vi "Write Sample Time.vi"(8 "error in (no error)":errorcluster, 10 "Sample Time":i32=1000, 11 "SensorInfo in":refnum<class "SensorInfo.lvclass">) -> (0 "error out":errorcluster, 3 "SensorInfo out":refnum<class "SensorInfo.lvclass">)   [LabVIEW 2012, in "Sensor Definition.lvlib" / "SensorInfo.lvclass"]
uses:
  SensorInfo.lvclass
  SensorInfo.lvclass/SensorInfo.ctl
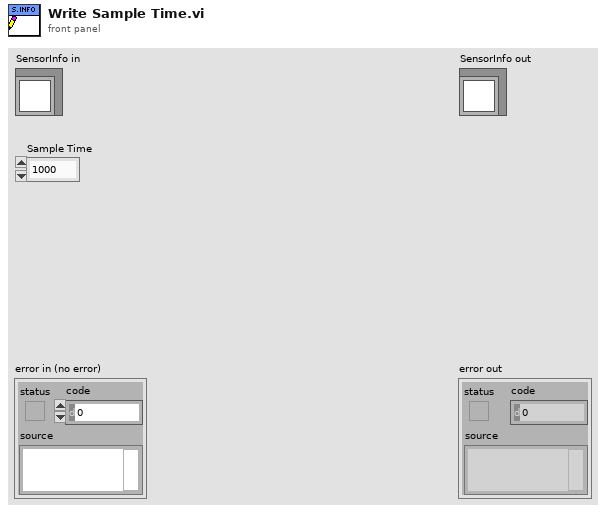
[diagram p1: front panel]
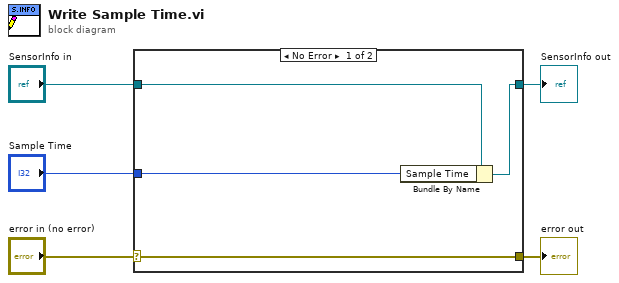
[diagram p0: block diagram]
diagram:
  n1 = case shown="No Error" "error in (no error)" {
    selector: "error in (no error)" -> [w9 w10]
    tunnel: [w9 w10] -> w4
    tunnel: [w7 w11] -> w2
    tunnel: "SensorInfo in" -> [w8 w11]
    tunnel: "Sample Time" -> [w6 _]
    frame No Error {
      n2 = Bundle By Name(cluster=w8, "Sample Time"=w6) -> (w7:refnum<class "SensorInfo.lvclass">)
    }
    frame Error {
    }
  }
  "error out" <- w4
  "SensorInfo out" <- w2
